vi "Get Routing Channel State-Value Table.vi"(8 "error in":errorcluster, 11 "routing channel in":T1 format="%.0x") -> (0 "error out":errorcluster, 1 "state values":i32[](array[numeric]), 2 "state names":string[](array[string]), 3 "routing channel out":T1=18446744073709551615 format="%.0x")   [LabVIEW 2020, in "Routing and Faulting Scripting.lvlib"]
doc: "Returns the names and values of the states for the routing channel."
uses:
  Routing and Faulting Scripting.lvlib
  <vilib>/NI VeriStand/Custom Device API/Custom Device Item Ref.ctl
  NationalInstruments.VeriStand.SystemDefinitionAPI
  NationalInstruments.VeriStand.SystemStorage
  Shared/Routing and Faulting Shared.lvlib
  <vilib>/NI VeriStand/Custom Device API/Custom Device API.lvlib
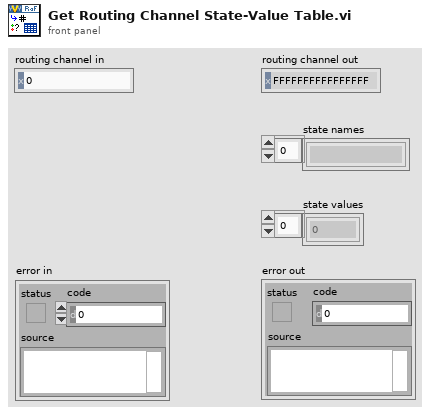
[diagram p1: front panel]
types:
  T1 = typedef "Custom Device API.lvlib/Custom Device Item Ref.ctl" = u64
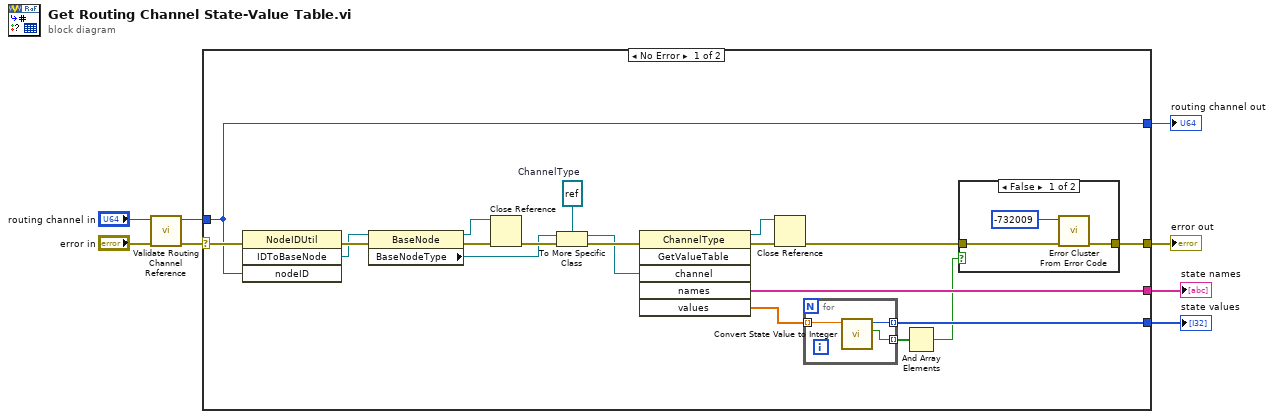
[diagram p0: block diagram]
diagram:
  n1 = call "Validate Routing Channel Reference.vi"("error in"="error in", "routing channel in"="routing channel in") -> ("error out"=w3:errorcluster, "routing channel out"=w1:T1)  [unwired: 8 in]
  n2 = case shown="No Error" w3 {
    selector: w3 -> [w25 w37]
    tunnel: [w9 w37] -> w7
    tunnel: w1 -> [w24 w36]
    tunnel: [w24 w36] -> w6
    tunnel: [w16 _] -> w5
    tunnel: [w13 _] -> w4
    frame No Error {
      w22 = refnum<k24> refnum  # ChannelType
      n3 = invoke class="NodeIDUtil" method="IDToBaseNode"(error in=w25, "nodeID"=w24) -> (error out=w28:errorcluster, "IDToBaseNode"=w26:refnum<k24>)  [unwired: 2 in, 2 out]
      n4 = property class="BaseNode"(reference=w26, error in=w28) -> (reference out=w15:refnum<k24>, error out=w27:errorcluster, "BaseNodeType"=w19:refnum<k24>)
      n5 = Close Reference(reference=w15, error in (no error)=w27) -> (error out=w20:errorcluster)
      n6 = To More Specific Class(target class=w22, reference=w19, error in=w20) -> (specific class reference=w21:refnum<k24>, error out=w23:errorcluster)
      n7 = invoke class="ChannelType" method="GetValueTable"(error in=w23, "channel"=w21) -> (reference out=w17:refnum<k24>, error out=w18:errorcluster, "names"=w16:string[], "values"=w14:dbl[])  [unwired: 4 in, 2 out]
      n8 = Close Reference(reference=w17, error in (no error)=w18) -> (error out=w10:errorcluster)
      n9 = for {
        tunnel: w14 -> [w35] mode=indexing
        tunnel: [w34] -> w13 mode=indexing
        tunnel: [w33] -> w12 mode=indexing
        n10 = call "Convert State Value to Integer.vi"("Floating Point State Value"=w35) -> ("Valid State Value"=w33:bool, "Integer State Value"=w34:i32)  [unwired: 9 in]
      }
      n11 = And Array Elements(Boolean array=w12) -> (logical AND=w11:bool)
      n12 = case shown="False" w11 {
        tunnel: w10 -> [w31 w32]
        tunnel: [w30 w32] -> w9
        frame False {
          n13 = call <vilib>:"Error Cluster From Error Code.vi"("error in (no error)"=w31, "error code (0)"=-732009) -> ("error out"=w30:errorcluster)  [unwired: 7 in]
        }
        frame True {
        }
      }
    }
    frame Error {
    }
  }
  "routing channel out" <- w6
  "error out" <- w7
  "state names" <- w5
  "state values" <- w4
